vi "Read PDP Values.vi"() -> (3 "all currents (A)":dbl[](array[numeric]))   [LabVIEW 2018]
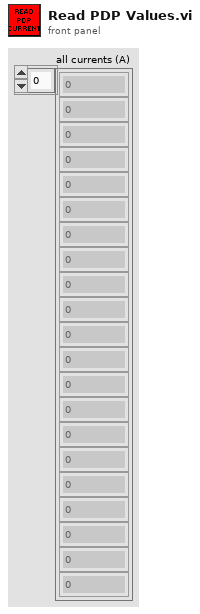
[diagram p1: front panel]
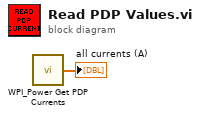
[diagram p0: block diagram]
diagram:
  n1 = call <vilib>:"WPI_Power Get PDP Currents.vi"() -> ("all currents (A)"=→"all currents (A)":dbl[])  [unwired: 13 in, 2 out]
